vi "VMI-Scan.vi"() -> ()   [LabVIEW 2018]
uses:
  <vilib>/Utility/file.llb/Write Delimited Spreadsheet (DBL).vi
panel:
  in  "File Name":string
  in  "Scan Number":string
  out "Progress Bar":dbl(slide) scale=0.0..100.0
  out "Time Remaining (min)":dbl
  out "Scan Time (min)":dbl
  in  "Gate Length 2":i32=1000
  in  "Gate Index 2":i32
  in  "Save Data?":bool=TRUE
  out "Timebase (ns)":u32
  in  "Scope Settings":T1={"VISA resource name"="Oscilloscope", "Signal Channel"=1, "Trigger Channel"=0, "Vertical Range (10.0 V)"=0.001, "Input Impedance (0: 1M ohm)"=1, "Acquisition Type (0:Sample)"=3, "Position (0.0 s)"=0.0, "Record Length (10000)"=1000, "Trigger Level (0.0V)"=1.0, "Average Waveforms (10)"=300} {"Acquisition Type (0:Sample)" items=["Sample", "Peak Detect", "Hi Res", "Average", "Envelope", "WfmDB"]; "Input Impedance (0: 1M ohm)" items=["1M", "50"]; "Trigger Channel" format="%#_5f" items=["Channel 1", "Channel 2", "Channel 3", "Channel 4", "Math 1", "Math 2", "Math 3", "Math 4", "Reference 1", "Reference 2", "Reference 3", "Reference 4"]; "Signal Channel" format="%#_5f" items=["Channel 1", "Channel 2", "Channel 3", "Channel 4", "Math 1", "Math 2", "Math 3", "Math 4", "Reference 1", "Reference 2", "Reference 3", "Reference 4"]}
  out "Full Waveform":waveform(dbl)(graph)={"t0"=timestamp(1.815305999999491e-07 s since 1904-01-01), "dt"=5e-07, "Y"=array[10000 elements]}
  out "Gate":dbl[](graph)
  in  "Setup Gate":bool
  in  "Directory Path":path=path "C:/Users/Cletus/Desktop/VMI Scan/100318"
  out "Step Number":i32
  out "REMPI Spectrum":cluster{"Y":dbl[], "Y":dbl[]}[](graph)=[{"Y"=[450.5], "Y"=[-0.0]}]
  out "Full Waveform":waveform(dbl)(graph)={"t0"=timestamp(1.815305999999491e-07 s since 1904-01-01), "dt"=5e-07, "Y"=array[10000 elements]}
  out "Gate":dbl[](graph)
  out "Gate Start (ns)":dbl
  out "Gate Length (ns)":dbl
  out "Sum of Intensity (V)":dbl
  in  "Gate Length":i32=40
  in  "Gate Index":i32=440
  out "Timebase (ns)":u32
  in  "Scope Settings":T2={"Scope Port (Scope)"="Oscilloscope", "Signal Channel"=1, "Trigger Channel"=0, "Vertical Range (10.0 V)"=0.001, "Input Impedance (0: 1M ohm)"=1, "Acquisition Type (0:Sample)"=3, "Position (0.0 s)"=0.0, "Record Length (10000)"=1000, "Trigger Level (0.0V)"=1.0, "Average Waveforms (10)"=30} {"Acquisition Type (0:Sample)" items=["Sample", "Peak Detect", "Hi Res", "Average", "Envelope", "WfmDB"]; "Input Impedance (0: 1M ohm)" items=["1M", "50"]; "Trigger Channel" format="%#_5f" items=["Channel 1", "Channel 2", "Channel 3", "Channel 4", "Math 1", "Math 2", "Math 3", "Math 4", "Reference 1", "Reference 2", "Reference 3", "Reference 4"]; "Signal Channel" format="%#_5f" items=["Channel 1", "Channel 2", "Channel 3", "Channel 4", "Math 1", "Math 2", "Math 3", "Math 4", "Reference 1", "Reference 2", "Reference 3", "Reference 4"]}
  out "Number of Steps":dbl
  in  "Scan":bool
  in  "Step Size":dbl=0.01 format="%#_13g"
  in  "Initial WL":dbl=259.5 format="%.2f"
  in  "Final WL":dbl=270.0 format="%.2f"
  out "Current WL (cm-1)":dbl
  out "Current WL (nm)":dbl format="%.2f"
  out "New WL (nm)":dbl format="%.2f"
  out "New WL (cm-1)":dbl
  in  "Change WL (nm) to:":dbl format="%.2f"
  in  "Change WL":bool
  in  "Laser Port (Laser)":refnum<visa-resource-name>="Laser"
  out "nm":dbl format="%.2f"
  out "cm-1":dbl format="%#_7g"
  in  "Check Current WL":bool
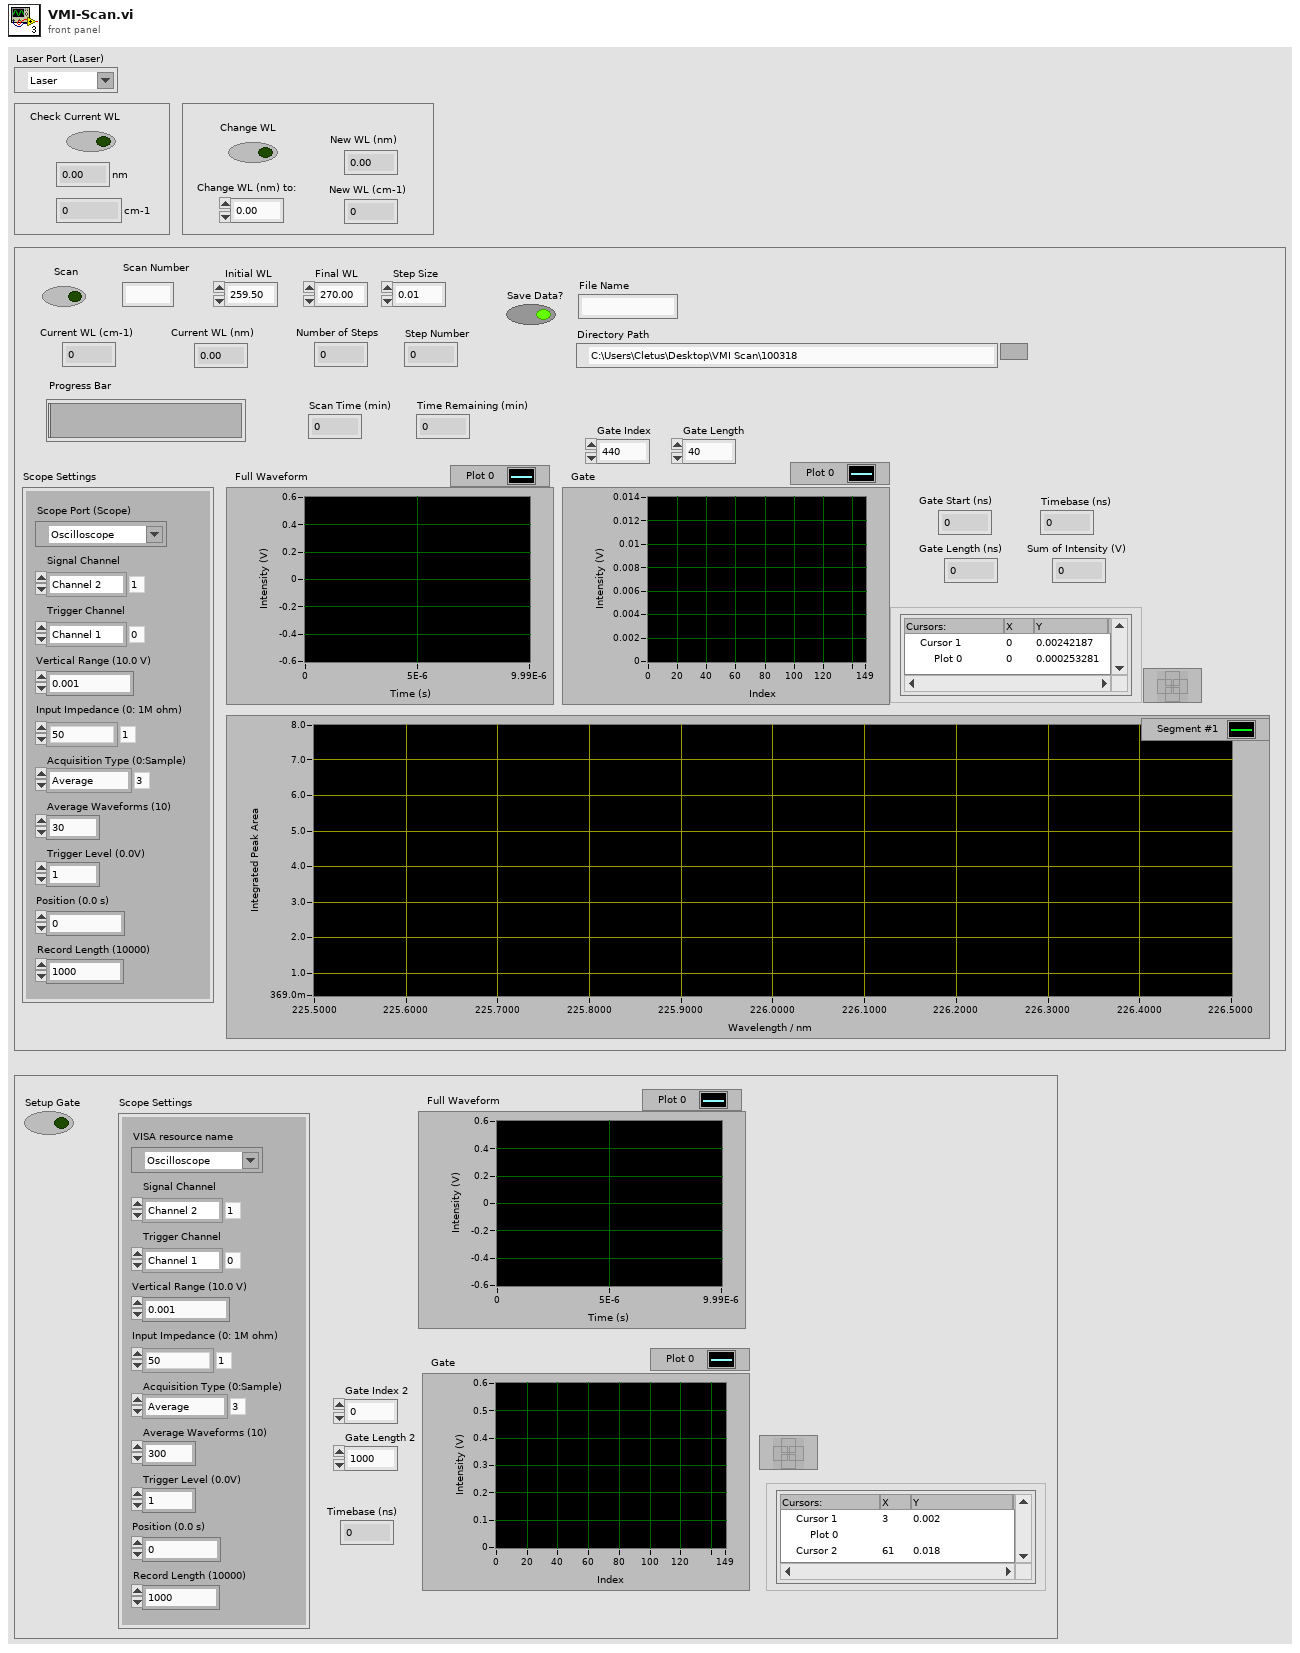
[diagram p1: front panel]
types:
  T1 = cluster{"VISA resource name":refnum<visa-resource-name>, "Signal Channel":u16, "Trigger Channel":u16, "Vertical Range (10.0 V)":dbl, "Input Impedance (0: 1M ohm)":u16, "Acquisition Type (0:Sample)":u16, "Position (0.0 s)":dbl, "Record Length (10000)":u32, "Trigger Level (0.0V)":dbl, "Average Waveforms (10)":i32}
  T2 = cluster{"Scope Port (Scope)":refnum<visa-resource-name>, "Signal Channel":u16, "Trigger Channel":u16, "Vertical Range (10.0 V)":dbl, "Input Impedance (0: 1M ohm)":u16, "Acquisition Type (0:Sample)":u16, "Position (0.0 s)":dbl, "Record Length (10000)":u32, "Trigger Level (0.0V)":dbl, "Average Waveforms (10)":i32}
  T3 = enum16{"open", "replace", "create", "open or create", "replace or create", "replace or create with confirmation"}
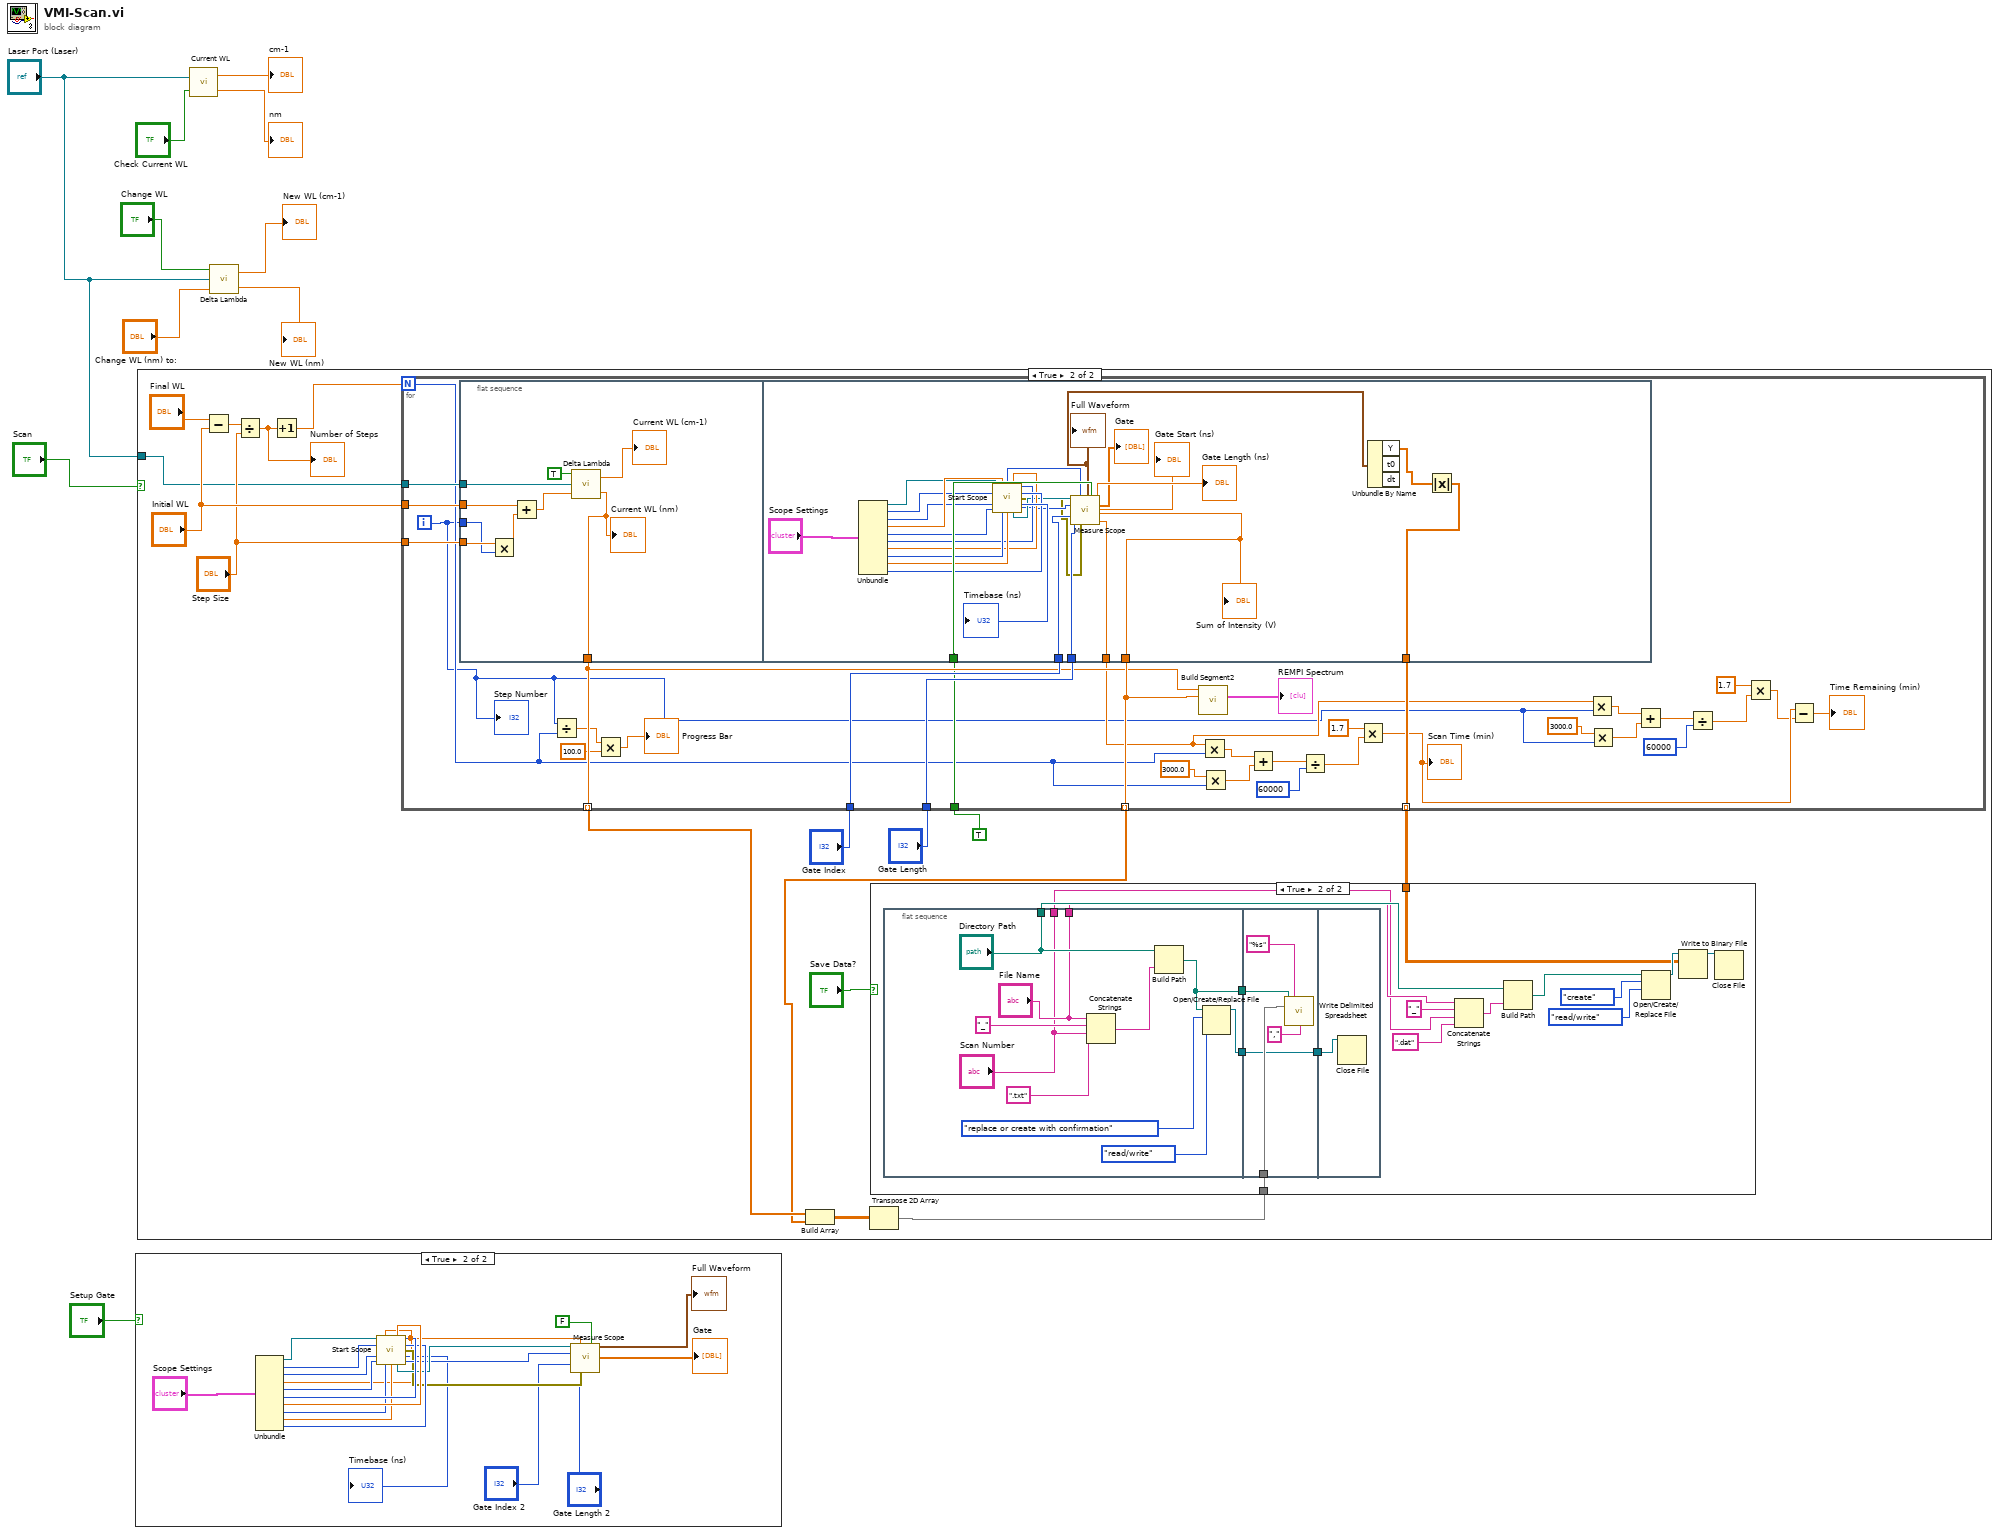
[diagram p0: block diagram]
diagram:
  n1 = case shown="True" "Setup Gate" {
    frame False {
    }
    frame True {
      n2 = Unbundle("Scope Settings") -> ("VISA resource name"=w27:refnum<visa-resource-name>, "Signal Channel"=w26:u16, "Trigger Channel"=w25:u16, "Vertical Range (10.0 V)"=w15:dbl, "Input Impedance (0: 1M ohm)"=w24:u16, "Acquisition Type (0:Sample)"=w23:u16, "Position (0.0 s)"=w22:dbl, "Record Length (10000)"=w21:u32, "Trigger Level (0.0V)"=w20:dbl, "Average Waveforms (10)"=w19:i32)
      n3 = call "Start Scope.vi"("VISA resource name"=w27, "Vertical Range (10.0 V)"=w15, "Position (0.0 s)"=w22, "Acquisition Type (0:Sample)"=w23, "Signal Channel"=w26, "Average Waveforms (10)"=w19, "Trigger Channel"=w25, "Input Impedance (0: 1M ohm)"=w24, "Record Length (10000)"=w21, "Trigger Level (0.0V)"=w20) -> ("error out"=w16:errorcluster, "Timebase"=→"Timebase (ns)":u32, "VISA resource name out"=w18:refnum<visa-resource-name>, "Signal Channel \nOut"=w17:u16)  [unwired: 1 in, 1 out]
      n4 = call "Measure Scope.vi"("VISA resource name"=w18, "Avg Num Samples"=w15, "Boolean"=FALSE, "Channel1 (0:Channel1)"=w17, "Gate Index"="Gate Index 2", "Gate Length"="Gate Length 2", "error in (no error)"=w16) -> ("Full Waveform"=→"Full Waveform":waveform(dbl), "Gate"=→"Gate":dbl[])  [unwired: 3 in, 4 out]
    }
  }
  n5 = case shown="True" "Scan" {
    tunnel: "Laser Port (Laser)" -> [_ w42]
    frame False {
    }
    frame True {
      n6 = Subtract(x="Final WL", y="Initial WL") -> (x-y=w44:dbl)
      n7 = Divide(x=w44, y="Step Size") -> (x/y=w31:dbl)
      "Number of Steps" <- w31
      n8 = Increment(x=w31) -> (x+1=w41:dbl)
      n9 = for {
        N: w41 -> [w83]
        tunnel: w42 -> [w111]
        tunnel: "Step Size" -> [w110]
        tunnel: "Initial WL" -> [w109]
        tunnel: [w105] -> w38 mode=indexing
        tunnel: "Gate Index" -> [w108]
        tunnel: "Gate Length" -> [w107]
        tunnel: [w106] -> w37 mode=indexing
        tunnel: TRUE ("Boolean") -> [w103]
        tunnel: [w102] -> w32 mode=indexing
        i -> [w82]
        n10 = flat-sequence {
          tunnel: w111 -> [w120]
          tunnel: w110 -> [w119]
          tunnel: w82 -> [w117]
          tunnel: w109 -> [w116]
          tunnel: [w112] -> w105
          tunnel: w108 -> [w147]
          tunnel: w107 -> [w146]
          tunnel: [w121] -> w106
          tunnel: w103 -> [w142]
          tunnel: [w122] -> w102
          tunnel: [w124] -> w88
          frame #0 {
            n11 = Multiply(x=w119, y=w117) -> (x*y=w118:dbl)
            n12 = Add(x=w116, y=w118) -> (x+y=w115:dbl)
            n13 = call "Delta Lambda.vi"("Change Lambda (nm) to:"=w115, "COM4"=w120, "Boolean"=TRUE) -> ("New Lambda (nm)"=w112:dbl, "New Lambda (cm-1)"=→"Current WL (cm-1)":dbl)
            "Current WL (nm)" <- w112
          }
          frame #1 {
            n14 = Unbundle("Scope Settings") -> ("Scope Port (Scope)"=w131:refnum<visa-resource-name>, "Signal Channel"=w132:u16, "Trigger Channel"=w133:u16, "Vertical Range (10.0 V)"=w134:dbl, "Input Impedance (0: 1M ohm)"=w135:u16, "Acquisition Type (0:Sample)"=w136:u16, "Position (0.0 s)"=w137:dbl, "Record Length (10000)"=w138:u32, "Trigger Level (0.0V)"=w139:dbl, "Average Waveforms (10)"=w140:i32)
            n15 = call "Start Scope.vi"("VISA resource name"=w131, "Vertical Range (10.0 V)"=w134, "Position (0.0 s)"=w137, "Acquisition Type (0:Sample)"=w136, "Signal Channel"=w132, "Average Waveforms (10)"=w140, "Trigger Channel"=w133, "Input Impedance (0: 1M ohm)"=w135, "Record Length (10000)"=w138, "Trigger Level (0.0V)"=w139) -> ("Average Waveforms (10) Out"=w129:i32, "error out"=w126:errorcluster, "Timebase"=→"Timebase (ns)":u32, "VISA resource name out"=w128:refnum<visa-resource-name>, "Signal Channel \nOut"=w127:u16)  [unwired: 1 in]
            n16 = call "Measure Scope.vi"("VISA resource name"=w128, "Avg Num Samples"=w129, "Boolean"=w142, "Channel1 (0:Channel1)"=w127, "Gate Index"=w147, "Gate Length"=w146, "error in (no error)"=w126) -> ("Full Waveform"=w125:waveform(dbl), "Gate"=→"Gate":dbl[], "Signal Duration (ns)"=→"Gate Length (ns)":dbl, "Signal Arrival (ns)"=→"Gate Start (ns)":dbl, "Sum of Intensity (V)"=w121:dbl, "Wait Time (ms)"=w124:dbl)  [unwired: 3 in]
            "Sum of Intensity (V)" <- w121
            "Full Waveform" <- w125
            n17 = Unbundle By Name(w125) -> ("Y"=w123:dbl[])  [unwired: 2 out]
            n18 = Absolute Value(x=w123) -> (abs(x)=w122:dbl[])
          }
        }
        n19 = Divide(x=w82, y=w83) -> (x/y=w80:dbl)
        n20 = Multiply(x=w80, y=100.0) -> (x*y=→"Progress Bar":dbl)
        n21 = call "Build Segment2"("Y Input"=w106, "X Input"=w105) -> ("XY Graph"=→"REMPI Spectrum":cluster{"Y":dbl[], "Y":dbl[]}[])  [unwired: 8 in, 1 out]
        n22 = Multiply(x=w88, y=w83) -> (x*y=w100:dbl)
        n23 = Multiply(x=3000.0, y=w83) -> (x*y=w99:dbl)
        n24 = Add(x=w100, y=w99) -> (x+y=w98:dbl)
        n25 = Divide(x=w98, y=u32 60000) -> (x/y=w95:dbl)
        n26 = Multiply(x=1.7, y=w95) -> (x*y=w86:dbl)
        "Scan Time (min)" <- w86
        n27 = Multiply(x=w88, y=w82) -> (x*y=w93:dbl)
        n28 = Multiply(x=3000.0, y=w82) -> (x*y=w92:dbl)
        n29 = Add(x=w93, y=w92) -> (x+y=w87:dbl)
        n30 = Divide(x=w87, y=u32 60000) -> (x/y=w89:dbl)
        n31 = Multiply(x=1.7, y=w89) -> (x*y=w85:dbl)
        n32 = Subtract(x=w86, y=w85) -> (x-y=→"Time Remaining (min)":dbl)
        "Step Number" <- w82
      }
      n33 = Build Array(w38, w37) -> (w36:dbl[][])
      n34 = Transpose 2D Array(2D array=w36) -> (transposed array=w35:dbl[][])
      n35 = case shown="True" "Save Data?" {
        tunnel: w35 -> [_ w59]
        tunnel: w32 -> [_ w52]
        frame False {
        }
        frame True {
          n36 = flat-sequence {
            tunnel: [w71] -> w62
            tunnel: [w69] -> w61
            tunnel: ["Directory Path"] -> w53
            tunnel: ["File Name"] -> w49
            tunnel: ["Scan Number"] -> w48
            tunnel: w62 -> [w77]
            tunnel: w59 -> [w75]
            tunnel: [w73] -> w60
            tunnel: w61 -> [w73]
            tunnel: w60 -> [w78]
            frame #0 {
              n37 = Concatenate Strings("File Name", "_" ("string"), "Scan Number", ".txt" ("string")) -> (w65:string)
              n38 = Build Path(base path="Directory Path", name or relative path=w65) -> (appended path=w71:path)
              n39 = Open/Create/Replace File(file path (use dialog)=w71, operation (0:open)=T3."replace or create with confirmation", access (0:read/write)=enum16{"read/write", "read-only", "write-only"}."read/write") -> (refnum out=w69:refnum<file>)  [unwired: 3 in, 2 out]
            }
            frame #1 {
              n40 = call-poly <vilib>:"Write Delimited Spreadsheet.vi"("file path (dialog if empty)"=w77, "format (%.3f)"="%s", "2D data"=w75, "delimiter (\\t)"="," ("delimiter (\\t)")) -> ()  [unwired: 10 in, 2 out]
            }
            frame #2 {
              n41 = Close File(refnum=w78) -> ()  [unwired: 1 in, 2 out]
            }
          }
          n42 = Concatenate Strings(w49, "_" ("string"), w48, ".dat" ("string")) -> (w47:string)
          n43 = Build Path(base path=w53, name or relative path=w47) -> (appended path=w56:path)
          n44 = Open/Create/Replace File(file path (use dialog)=w56, operation (0:open)=T3."create", access (0:read/write)=enum16{"read/write", "read-only", "write-only"}."read/write") -> (refnum out=w57:refnum<file>)  [unwired: 3 in, 2 out]
          n45 = Write to Binary File(file (use dialog)=w57, data=w52) -> (refnum out=w58:refnum<file>)  [unwired: 4 in, 2 out]
          n46 = Close File(refnum=w58) -> ()  [unwired: 1 in, 2 out]
        }
      }
    }
  }
  n47 = call "Current WL.vi"("Boolean"="Check Current WL", "VISA resource name"="Laser Port (Laser)") -> ("nm"=→"nm":dbl, "cm-1"=→"cm-1":dbl)
  n48 = call "Delta Lambda.vi"("Change Lambda (nm) to:"="Change WL (nm) to:", "COM4"="Laser Port (Laser)", "Boolean"="Change WL") -> ("New Lambda (nm)"=→"New WL (nm)":dbl, "New Lambda (cm-1)"=→"New WL (cm-1)":dbl)
